vi "Memory.Pointer.Read.Safe.1D.Bool.vi"(8 "error in (no error)":errorcluster, 9 "count":u64 format="%d elements", 10 "buffer in":bool[](array[boolean]), 11 "pointer in":refnum<class "Memory.Pointer.lvclass">) -> (0 "error out":errorcluster, 1 "count out":u64 format="%d elements", 2 "buffer out":bool[](array[boolean]), 3 "pointer out":refnum<class "Memory.Pointer.lvclass">)   [LabVIEW 2016, in "Memory Manager.lvlib" / "Memory.Pointer.lvclass"]
doc: "Reads the <b>count</b> elements of the specified data type from the address specified by <b>pointer</b> into the provided <b>buffer</b>.\n\n<b>Note:</b> This VI is <b>safe</b>.\n\nSafe means that this function evaluates the size parameter of <b>pointer</b> to ensure that is inbounds of allocated memory before peforming a memory read/write. Reading/writing more data to a pointer than it has allocated can corrupt or crash LabVIEW."
uses:
  Memory.Pointer.lvclass
  Memory.Pointer.lvclass/Memory.Pointer.ctl
  Accessors/Get Address.vi
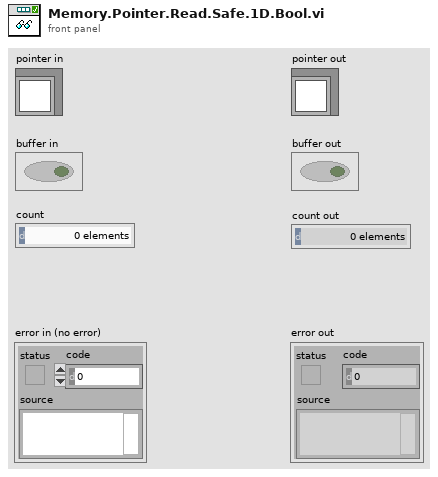
[diagram p1: front panel]
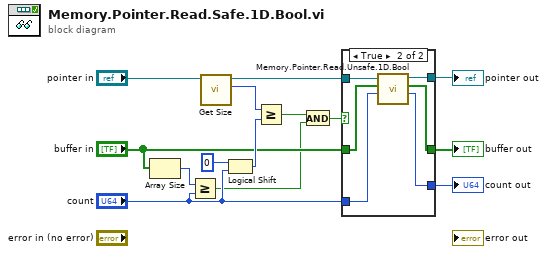
[diagram p0: block diagram]
diagram:
  n1 = Array Size(array="buffer in") -> (size(s)=w5:i32)
  n2 = Greater Or Equal?(x=w5, y="count") -> (x >= y?=w1:bool)
  n3 = call "Get Size.vi"("Pointer in"="pointer in") -> ("size"=w12:u64, "Pointer out"=w10:refnum<class "Memory.Pointer.lvclass">)  [unwired: 8 in, 1 out]
  n4 = Logical Shift(y=i16 0, x="count") -> (x << y=w11:u64)
  n5 = Greater Or Equal?(x=w12, y=w11) -> (x >= y?=w2:bool)
  n6 = And(x=w2, y=w1) -> (x .and. y?=w3:bool)
  n7 = case shown="True" w3 {
    tunnel: w10 -> [w17 w23]
    tunnel: [w17 w22] -> w9
    tunnel: [w16 w21] -> w8
    tunnel: "count" -> [w15 w20]
    tunnel: "buffer in" -> [w16 w19]
    tunnel: [w15 w18] -> w7
    frame False {
    }
    frame True {
      n8 = call "Memory.Pointer.Read.Unsafe.1D.Bool.vi"("count"=w20, "buffer in"=w19, "pointer in"=w23) -> ("count out"=w18:u64, "buffer out"=w21:bool[], "pointer out"=w22:refnum<class "Memory.Pointer.lvclass">)  [unwired: 5 in, 1 out]
    }
  }
  "pointer out" <- w9
  "buffer out" <- w8
  "count out" <- w7
